vi "SpectrumNormalOrdB.vi"(9 "20/10":bool, 10 "Normal/dB":bool, 11 "Spectras-Analiza":cluster{dbl[], dbl[]}[](array[cluster])) -> (2 "Spectras-Analiza":cluster{dbl[], dbl[]}[](array[cluster]))   [LabVIEW 2020]
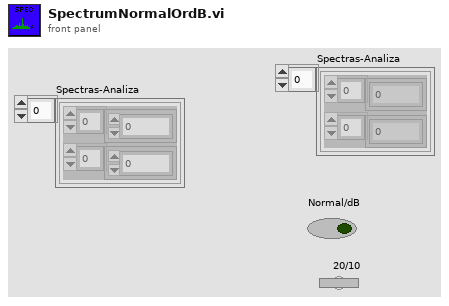
[diagram p1: front panel]
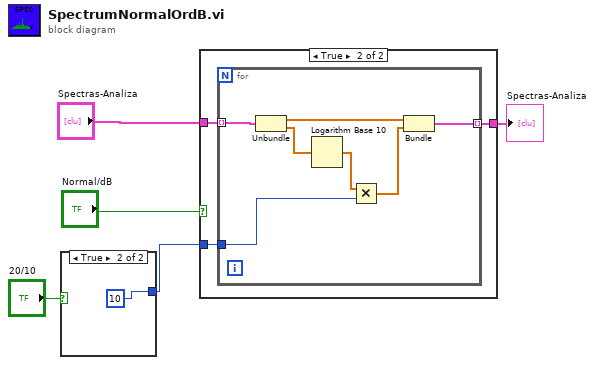
[diagram p0: block diagram]
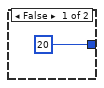
[diagram p2: hidden frame]
diagram:
  n1 = case shown="True" "20/10" {
    tunnel: [20 10] -> w2
    frame False {
    }
    frame True {
    }
  }
  n2 = case shown="True" "Normal/dB" {
    tunnel: "Spectras-Analiza" -> [w8 w11]
    tunnel: [w8 w10] -> w4
    tunnel: w2 -> [_ w9]
    frame False {
    }
    frame True {
      n3 = for {
        tunnel: w11 -> [w18] mode=indexing
        tunnel: [w13] -> w10 mode=indexing
        tunnel: w9 -> [w12]
        n4 = Unbundle(w18) -> (w15:dbl[], w17:dbl[])
        n5 = Logarithm Base 10(1:w17) -> (0:w16:dbl[])
        n6 = Multiply(x=w16, y=w12) -> (x*y=w14:dbl[])
        n7 = Bundle(w15, w14) -> (w13:cluster{dbl[], dbl[]})  [unwired: 1 in]
      }
    }
  }
  "Spectras-Analiza" <- w4
